vi "Alarm and Error Result.vi"(10 "Command":string) -> (2 "Alarm or Error":bool)   [LabVIEW 2017]
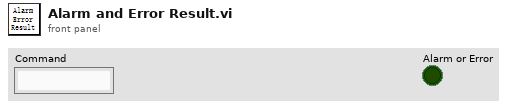
[diagram p1: front panel]
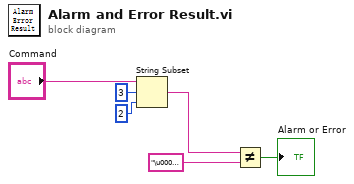
[diagram p0: block diagram]
diagram:
  n1 = String Subset(string="Command", offset (0)=3 ("偏移量(0)"), length (rest)=2 ("长度（剩余）")) -> (substring=w3:string)
  n2 = Not Equal?(x=w3, y="\u0000\u0000" ("子字符串")) -> (x != y?=→"Alarm or Error":bool)
